vi "Update inventory.vi"(8 "error in (no error)":errorcluster, 10 "Producto del inventario":i32, 11 "Soda Actors in":refnum<class "Soda Actors.lvclass">) -> (0 "error out":errorcluster, 3 "Soda Actors out":refnum<class "Soda Actors.lvclass">)   [LabVIEW 2020, in "Soda Actors.lvlib" / "Soda Actors.lvclass"]
uses:
  Soda Actors.lvclass
  Soda Actors.lvclass/Soda Actors.ctl
  <vilib>/Utility/config.llb/Read Key (Double).vi
  <vilib>/Utility/config.llb/Write Key (String).vi
  <vilib>/Utility/config.llb/Read Key (String).vi
  <vilib>/Utility/config.llb/NI_LVConfig.lvlib
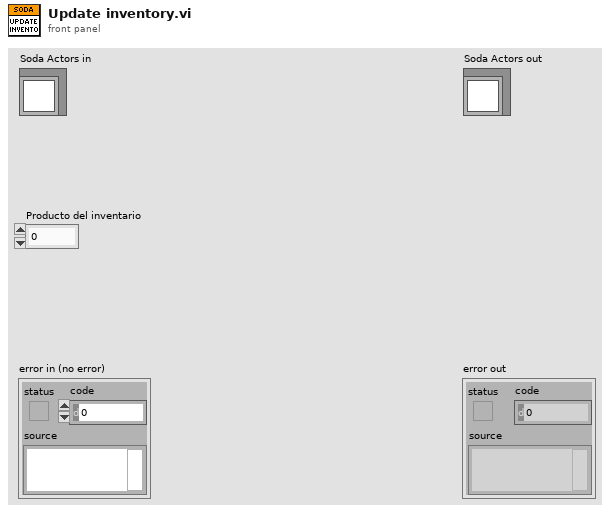
[diagram p1: front panel]
types:
  T1 = typedef "NI_LVConfig.lvlib/Config Data RefNum.ctl" = refnum<k1>
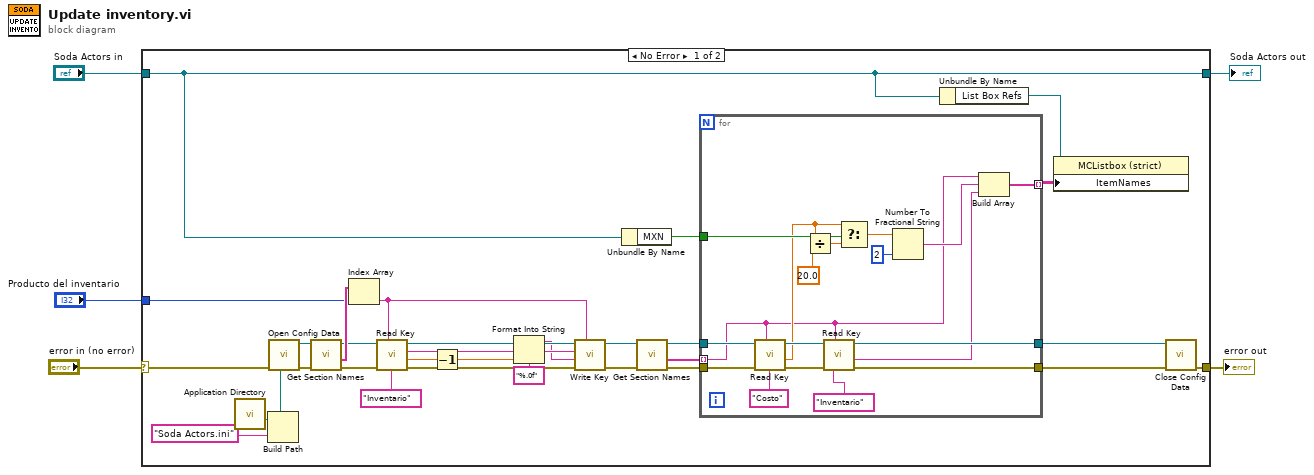
[diagram p0: block diagram]
diagram:
  n1 = case shown="No Error" "error in (no error)" {
    selector: "error in (no error)" -> [w23 w55]
    tunnel: [w22 w55] -> w4
    tunnel: [w12 w54] -> w2
    tunnel: "Soda Actors in" -> [w12 w54]
    tunnel: "Producto del inventario" -> [w32 _]
    frame No Error {
      w28 = "Inventario" ("key")
      n2 = call <vilib>:"Application Directory.vi"() -> ("Application Directory"=w8:path)
      n3 = Build Path(base path=w8, name or relative path="Soda Actors.ini" ("string")) -> (appended path=w6:path)
      n4 = call <vilib>:"Open Config Data.vi"("error in (no error)"=w23, "configuration file path"=w6) -> ("error out"=w35:errorcluster, "refnum"=w34:T1)  [unwired: 7 in, 1 out]
      n5 = call <vilib>:"Get Section Names.vi"("error in (no error)"=w35, "refnum"=w34) -> ("error out"=w31:errorcluster, "section names"=w33:string[], "refnum out"=w26:T1)  [unwired: 7 in]
      n6 = Index Array(array=w33, index=w32) -> (element=w25:string)
      n7 = call-poly <vilib>:"Read Key.vi"("section"=w25, "error in (no error)"=w31, "key"=w28, "refnum"=w26) -> ("error out"=w30:errorcluster, "value"=w29:dbl, "refnum out"=w27:T1)  [unwired: 4 in, 1 out]
      n8 = Decrement(x=w29) -> (x-1=w21:dbl)
      n9 = Format Into String(format string="%.0f", w21) -> (resulting string=w19:string)  [unwired: 2 in, 1 out]
      n10 = call-poly <vilib>:"Write Key.vi"("section"=w25, "error in (no error)"=w30, "value"=w19, "key"=w28, "refnum"=w27) -> ("error out"=w24:errorcluster, "refnum out"=w15:T1)  [unwired: 4 in, 1 out]
      n11 = Unbundle By Name(w12) -> ("MXN"=w11:bool)
      n12 = call <vilib>:"Get Section Names.vi"("error in (no error)"=w24, "refnum"=w15) -> ("error out"=w16:errorcluster, "section names"=w13:string[], "refnum out"=w14:T1)  [unwired: 7 in]
      n13 = for {
        tunnel: w14 -> [w51]
        tunnel: [w47] -> w17
        tunnel: w16 -> [w53]
        tunnel: [w49] -> w18
        tunnel: w13 -> [w36] mode=indexing
        tunnel: w11 -> [w43]
        tunnel: [w45] -> w9 mode=indexing
        n14 = call-poly <vilib>:"Read Key.vi"("section"=w36, "error in (no error)"=w53, "key"="Costo", "refnum"=w51) -> ("error out"=w52:errorcluster, "value"=w41:dbl, "refnum out"=w48:T1)  [unwired: 4 in, 1 out]
        n15 = Divide(x=w41, y=20.0) -> (x/y=w42:dbl)
        n16 = call-poly <vilib>:"Read Key.vi"("section"=w36, "error in (no error)"=w52, "key"="Inventario", "refnum"=w48) -> ("error out"=w49:errorcluster, "value"=w44:string, "refnum out"=w47:T1)  [unwired: 4 in, 1 out]
        n17 = Select(t=w41, s=w43, f=w42) -> (s? t:f=w39:dbl)
        n18 = Number To Fractional String(number=w39, precision (6)=i16 2) -> (F-format string=w37:string)  [unwired: 2 in]
        n19 = Build Array(w36, w37, w44) -> (w45:string[])
      }
      n20 = Unbundle By Name(w12) -> ("List Box Refs"=w10:refnum<vi>)
      n21 = property class="MCListbox (strict)"(reference=w10, "ItemNames"=w9) -> ()  [unwired: 1 in, 2 out]
      n22 = call <vilib>:"Close Config Data.vi"("error in (no error)"=w18, "refnum"=w17) -> ("error out"=w22:errorcluster)  [unwired: 8 in, 1 out]
    }
    frame Error {
    }
  }
  "error out" <- w4
  "Soda Actors out" <- w2
